vi "PathDialog.vi"() -> (3 "Cancelled?":bool)   [LabVIEW 2020]
doc: "Use this template to create a dialog box with event handling."
uses:
  global/SettingVariable.vi
  <vilib>/Utility/config.llb/Read Key (Path).vi
  <vilib>/Utility/config.llb/NI_LVConfig.lvlib
panel:
  in  "DRWM path 2":path caption="DRWM下段修正因子："
  in  "DRWM path 1":path caption="DRWM上段修正因子："
  in  "data path":path caption="数据文件保存路径："
  in  "Cancel":bool
  in  "OK":bool
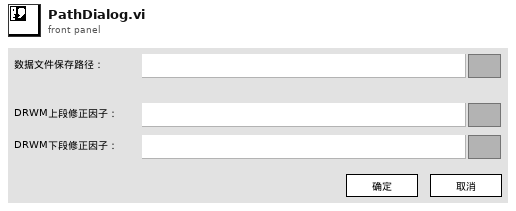
[diagram p1: front panel]
types:
  T1 = typedef "NI_LVConfig.lvlib/Config Data RefNum.ctl" = refnum<k1>
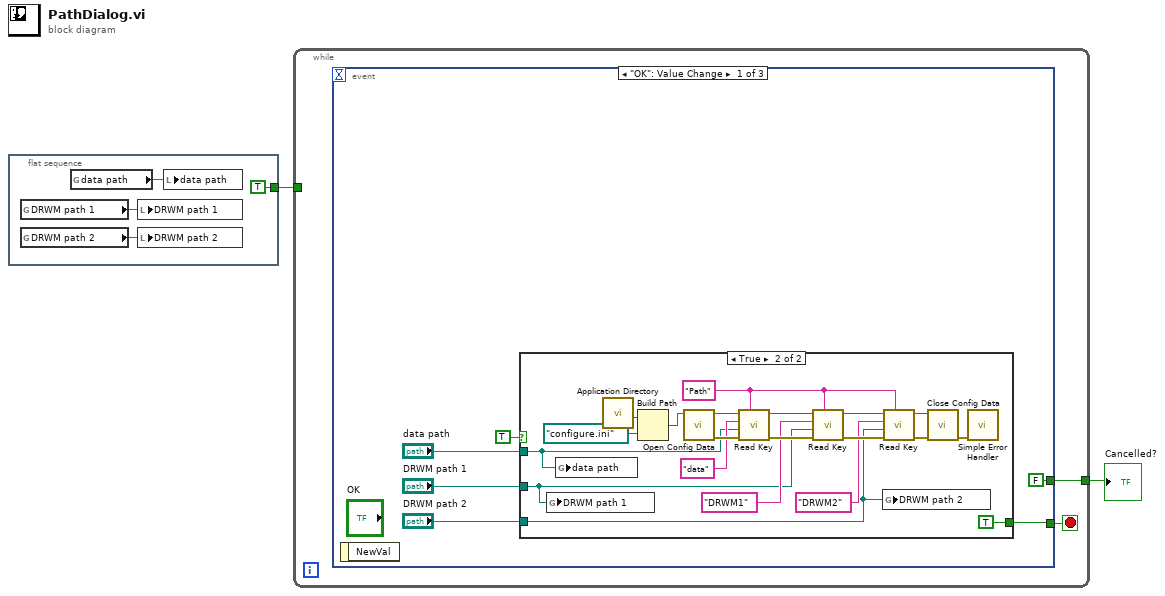
[diagram p0: block diagram]
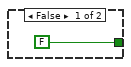
[diagram p2: hidden frame]
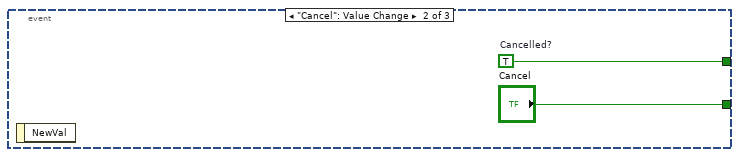
[diagram p3: hidden frame]
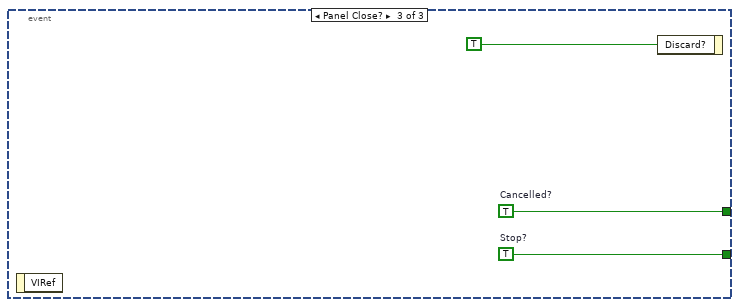
[diagram p4: hidden frame]
diagram:
  n1 = flat-sequence {
    tunnel: [TRUE] -> w1
    frame #0 {
      n2 = global read "SettingVariable.vi" "DRWM path 1"() -> (w5:path)
      n3 = global read "SettingVariable.vi" "DRWM path 2"() -> (w4:path)
      n4 = global read "SettingVariable.vi" "data path"() -> (w6:path)
      n5 = local write "DRWM path 1"(w5) -> ()
      n6 = local write "DRWM path 2"(w4) -> ()
      n7 = local write "data path"(w6) -> ()
    }
  }
  n8 = while {
    tunnel: [w7] -> w2
    tunnel: w1 -> [_]
    stop <- w8 stop-if-true
    n9 = event shown="[0] \"OK\": Value Change" {
      selector: _ -> [_ _ _]
      dyn-events: _ -> [_ _ _]
      timeout: _ -> [_ _ _]
      tunnel: [w12 "Cancel" w39] -> w8
      tunnel: [FALSE ("Cancelled?") w37 w38] -> w7
      event "OK": Value Change {
        n10 = event-data() -> ()  [unwired: 1 in, 1 out]
        n11 = case shown="True" TRUE {
          tunnel: [FALSE ("Stop?") TRUE ("Stop?")] -> w12
          tunnel: "data path" -> [_ w18]
          tunnel: "DRWM path 1" -> [_ w17]
          tunnel: "DRWM path 2" -> [_ w16]
          frame False {
          }
          frame True {
            w25 = "Path" ("section")
            n12 = global write "SettingVariable.vi" "DRWM path 1"(w17) -> ()
            n13 = global write "SettingVariable.vi" "data path"(w18) -> ()
            n14 = call <vilib>:"Application Directory.vi"() -> ("Application Directory"=w34:path)
            n15 = Build Path(base path=w34, name or relative path=path "configure.ini") -> (appended path=w32:path)
            n16 = call <vilib>:"Open Config Data.vi"("configuration file path"=w32) -> ("error out"=w30:errorcluster, "refnum"=w31:T1)  [unwired: 2 in, 7 out]
            n17 = call-poly <vilib>:"Read Key.vi"("section"=w25, "error in (no error)"=w30, "default value"=w18, "key"="data" ("section"), "refnum"=w31) -> ("error out"=w28:errorcluster, "refnum out"=w29:T1)  [unwired: 3 in, 2 out]
            n18 = call-poly <vilib>:"Read Key.vi"("section"=w25, "error in (no error)"=w28, "default value"=w17, "key"="DRWM1" ("section"), "refnum"=w29) -> ("error out"=w26:errorcluster, "refnum out"=w27:T1)  [unwired: 3 in, 2 out]
            n19 = global write "SettingVariable.vi" "DRWM path 2"(w16) -> ()
            n20 = call-poly <vilib>:"Read Key.vi"("section"=w25, "error in (no error)"=w26, "default value"=w16, "key"="DRWM2" ("section"), "refnum"=w27) -> ("error out"=w22:errorcluster, "refnum out"=w23:T1)  [unwired: 3 in, 2 out]
            n21 = call <vilib>:"Close Config Data.vi"("error in (no error)"=w22, "refnum"=w23) -> ("error out"=w24:errorcluster)  [unwired: 1 in, 8 out]
            n22 = call <vilib>:"Simple Error Handler.vi"("error in (no error)"=w24) -> ()  [unwired: 1 in, 8 out]
          }
        }
      }
      event "Cancel": Value Change {
        w37 = TRUE  # Cancelled?
        n23 = event-data() -> ()  [unwired: 1 in, 1 out]
      }
      event Panel Close? {
        w38 = TRUE  # Cancelled?
        w39 = TRUE  # Stop?
        n24 = event-data() -> ()  [unwired: 1 in, 1 out]
        n25 = event-data("Discard?"=TRUE) -> ()  [unwired: 1 in, 1 out]
      }
    }
  }
  "Cancelled?" <- w2
